vi "Begin.vi"(8 "error in":errorcluster) -> (0 "error out":errorcluster)   [LabVIEW 2019]
doc: "Called before other user functions, this VI is expected to open initial I/O refnums, load in file data, and do all program initialization. Notice that the <B>error out</B> terminal is simply used for data flow. Wiring it to other structures or subVIs ensures that this VI runs first."
uses:
  <vilib>/Rock Robotics/WPI/DriverStation/WPI_DriverStationRobotMode2.ctl
  <vilib>/Rock Robotics/WPI/ThirdParty/Phoenix-LabVIEW/Motor Controller/Controls/CTRE_Phoenix_MotorControl_ControlMode.ctl
  <vilib>/Rock Robotics/WPI/Solenoid/WPI_SolenoidChannel.ctl
  <vilib>/Rock Robotics/WPI/Joystick/WPI_JoystickDeviceEnum.ctl
  <vilib>/Rock Robotics/SystemInterfaces/DIO/FPGA_DIOPWMChannel.ctl
  <vilib>/Rock Robotics/SystemInterfaces/DIO/FPGA_DIOChannel.ctl
  <vilib>/Rock Robotics/WPI/ThirdParty/Phoenix-LabVIEW/Motor Controller/Controls/CTRE_Phoenix_MotorControl_FeedbackDevice.ctl
  <vilib>/Rock Robotics/WPI/SafetyOutput/WPI_SafetyOutputConfigMenu.ctl
  Robot Global Data.vi
  <vilib>/Rock Robotics/Network Tables/NT Write String Array.vi
  <vilib>/Rock Robotics/WPI/Solenoid/WPI_SolenoidOpenDouble.vi
  <vilib>/Rock Robotics/WPI/Switch/WPI_SwitchOpenLimit.vi
  <vilib>/Rock Robotics/WPI/MotorControl/WPI_MotorControlOpen SPARK.vi
  <vilib>/Rock Robotics/WPI/RobotDrive/WPI_RobotDriveOpen2MotorWithExistingMotors.vi
  <vilib>/Rock Robotics/WPI/MotorControl/WPI_MotorControlOpen VictorSP.vi
  <vilib>/Rock Robotics/WPI/RobotDrive/WPI_RobotDriveOpen2MotorWithTalon.vi
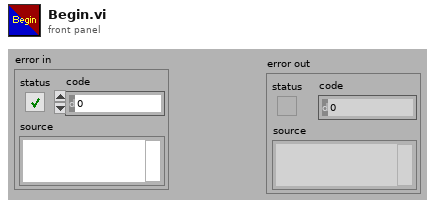
[diagram p1: front panel]
types:
  T1 = typedef "WPI_SafetyOutputConfigMenu.ctl" = enum16{"Enable", "Disable"}
  T2 = typedef "FPGA_DIOPWMChannel.ctl" = enum8{"PWM 0", "PWM 1", "PWM 2", "PWM 3", "PWM 4", "PWM 5", "PWM 6", "PWM 7", "PWM 8", "PWM 9", "PWM MXP 0", "PWM MXP 1", "PWM MXP 2", "PWM MXP 3", "PWM MXP 4", "PWM MXP 5", "PWM MXP 6", "PWM MXP 7", "PWM MXP 8", "PWM MXP 9", "Invalid"}
  T3 = typedef "WPI_JoystickDeviceEnum.ctl" = enum16{"USB 0", "USB 1", "USB 2", "USB 3", "USB 4", "USB 5"}
  T4 = typedef "CTRE_Phoenix_MotorControl_FeedbackDevice.ctl" = i8
  T5 = typedef "WPI_SolenoidChannel.ctl" = enum8{"Solenoid 0", "Solenoid 1", "Solenoid 2", "Solenoid 3", "Solenoid 4", "Solenoid 5", "Solenoid 6", "Solenoid 7", "Invalid"}
  T6 = typedef "CTRE_Phoenix_MotorControl_ControlMode.ctl" = u16
  T7 = typedef "FPGA_DIOChannel.ctl" = enum8{"DIO 0", "DIO 1", "DIO 2", "DIO 3", "DIO 4", "DIO 5", "DIO 6", "DIO 7", "DIO 8", "DIO 9", "DIO MXP 0", "DIO MXP 1", "DIO MXP 2", "DIO MXP 3", "DIO MXP 4", "DIO MXP 5", "DIO MXP 6", "DIO MXP 7", "DIO MXP 8", "DIO MXP 9", "DIO MXP 10", "DIO MXP 11", "DIO MXP 12", "DIO MXP 13", "DIO MXP 14", "DIO MXP 15", "SPI Port CS1", "SPI Port CS2", "SPI Port CS3", "SPI Port MISO", "SPI Port MOSI", "Invalid"}
  T8 = typedef "WPI_DriverStationRobotMode2.ctl" = enum16{"Autonomous Disabled", "Autonomous Enabled", "Teleop Disabled", "Teleop Enabled", "Disconnected", "Finish", "Test Disabled", "Test Enabled", "Emergency Stopped"}
  T9 = typedef "WPI_JoystickDevRef.ctl" = cluster{"Device":T3}
  T10 = typedef "WPI_RobotDriveDevRef.ctl" = cluster{"DevStatus":errorcluster, "Motors[]":T11[], "Square Inputs":bool, "Max Output":dbl}
  T11 = typedef "WPI_MotorControlDeviceRef.ctl" = cluster{"DeviceStatus":errorcluster, "Type":T12, "PWM":cluster{"PWM Channel":T2, "DeadBand":T13}, "CAN":cluster{"Device Number":u8, "SetOutput VI Ref":variant, "GetOutput VI Ref":variant, "Enable VI Ref":variant, "Disable VI Ref":variant, "Data":variant}, "Invert":bool, "DIO PWM":cluster{"PWM \"Enable\" Channel":T2, "DIOChannel":T7, "PWM Rate":dbl}}
  T12 = typedef "WPI_MotorControlType.ctl" = enum16{"PWM", "CAN", "DIO PWM"}
  T13 = typedef "WPI_PWMDeadband.ctl" = cluster{"Name":string, "maxPositivePwm":i32, "minPositivePwm":i32, "centerPwm":i32, "maxNegativePwm":i32, "minNegativePwm":i32, "angularRange":u16}
  T14 = typedef "WPI_ServoDeviceRef.ctl" = cluster{"DeviceStatus":errorcluster, "PWM Channel":T2, "DeadBand":T13}
  T15 = typedef "WPI_SwitchDevRef.ctl" = cluster{"DevStatus":errorcluster, "DIO Channel":T7, "CntIndex":T16, "Normally Closed":bool}
  T16 = typedef "FPGA_CounterCtrSystemIndex.ctl" = enum8{"Ctr 0", "Ctr 1", "Ctr 2", "Ctr 3", "Ctr 4", "Ctr 5", "Ctr 6", "Ctr 7", "Invalid"}
  T17 = typedef "WPI_SolenoidDevRef.ctl" = cluster{"DevStatus":errorcluster, "Pneumatics Control Module":u8, "Forward Solenoid Channel":T5, "Reverse Solenoid Channel":T5}
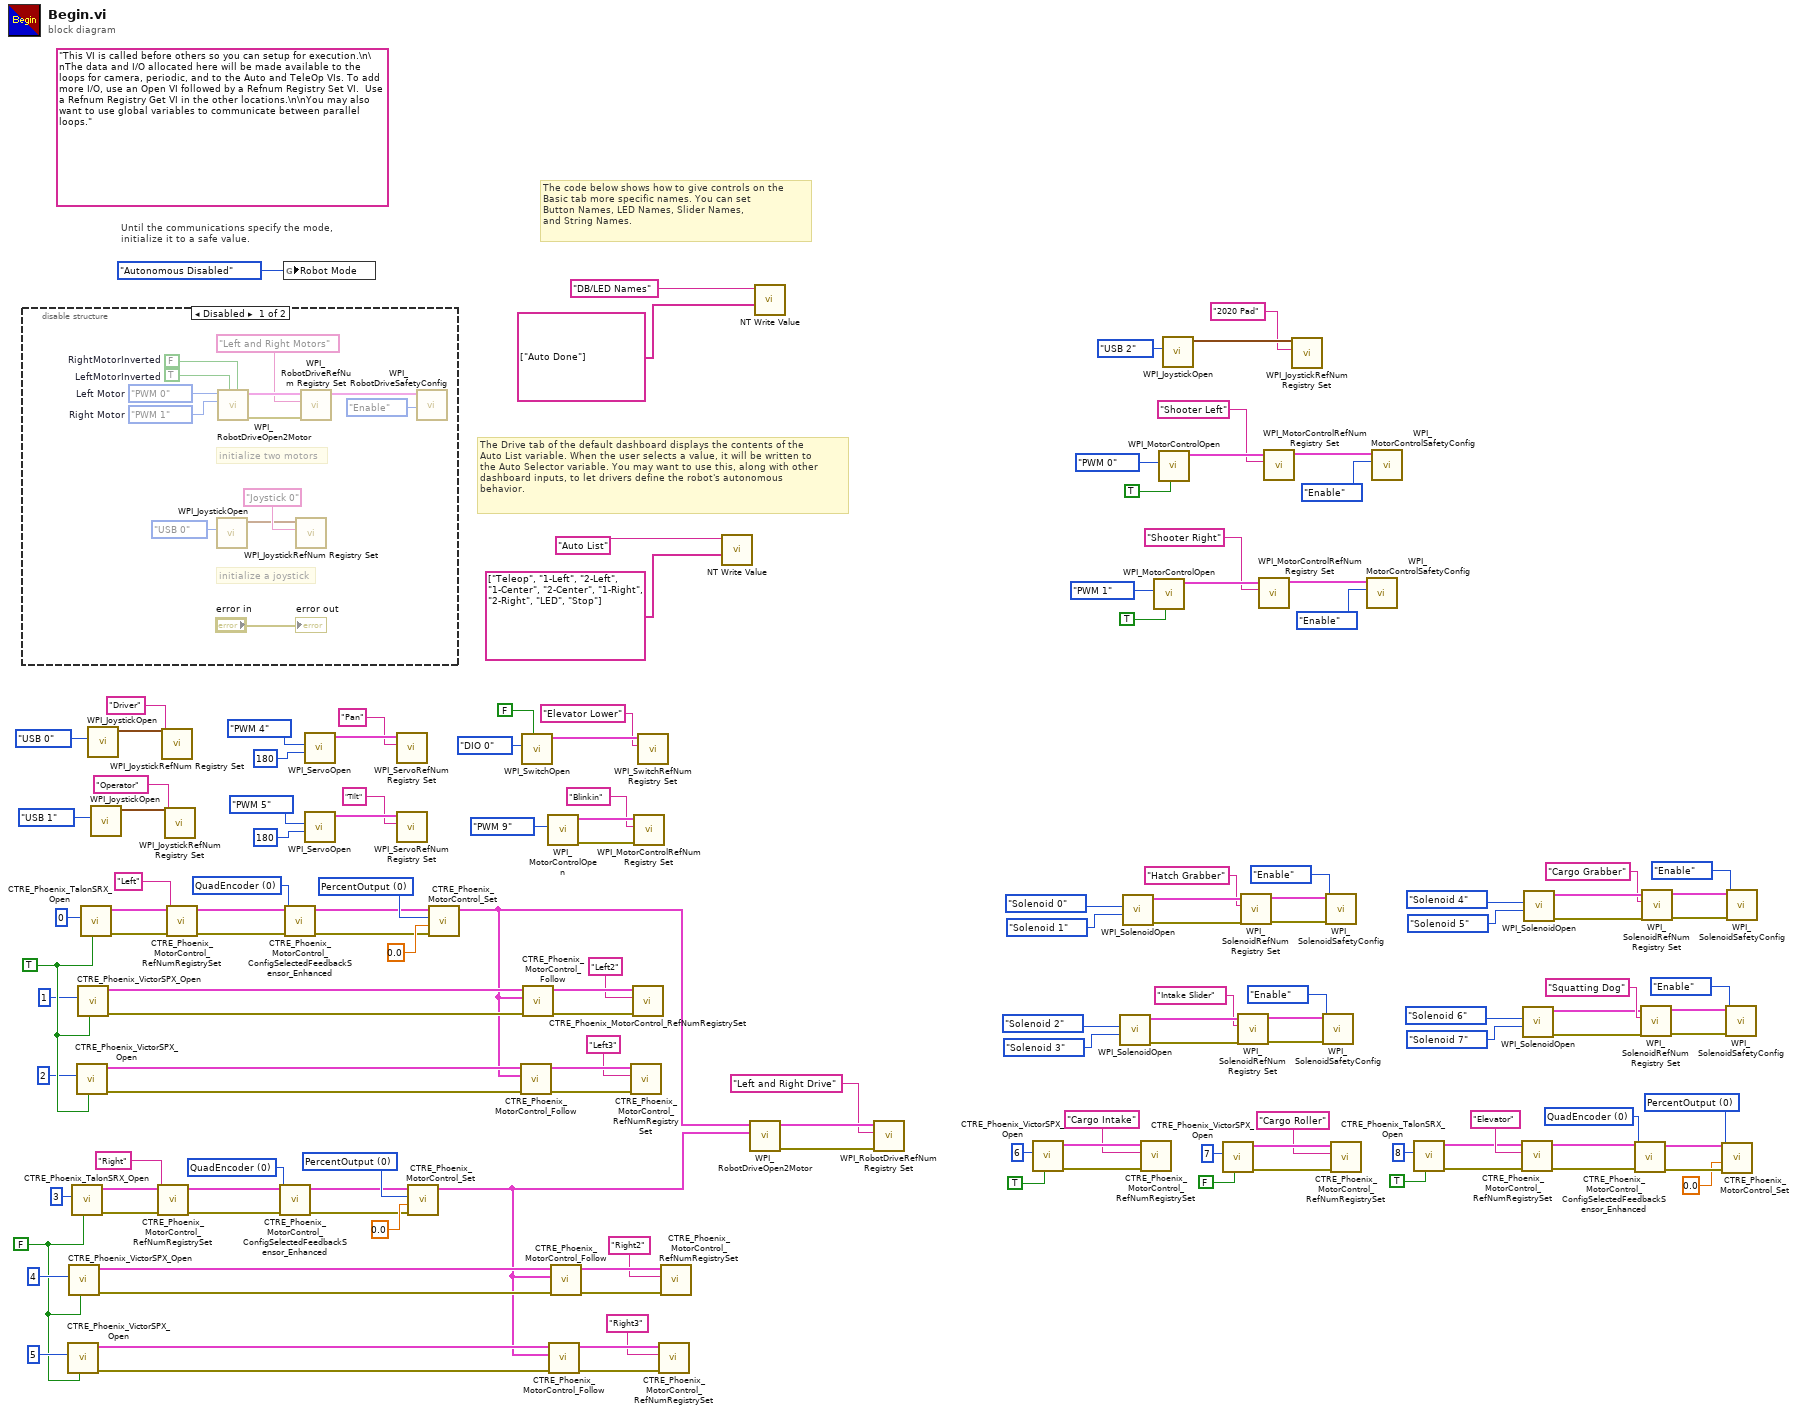
[diagram p0: block diagram]
diagram:
  w23 = T4 0 items=["QuadEncoder"=0, "Analog"=2, "Tachometer"=4, "Pulse Width Encoded Position"=8, "Sensor Sum (S0 + S1)"=9, "Sensor Difference (D0 - D1)"=10, "Remote Source 0"=11, "Remote Source 1"=12, "Software Emulated"=15] ("Feedback Device")
  w27 = T4 0 items=["QuadEncoder"=0, "Analog"=2, "Tachometer"=4, "Pulse Width Encoded Position"=8, "Sensor Sum (S0 + S1)"=9, "Sensor Difference (D0 - D1)"=10, "Remote Source 0"=11, "Remote Source 1"=12, "Software Emulated"=15] ("Feedback Device")
  w44 = T6 0 items=["PercentOutput"=0, "Position"=1, "Velocity"=2, "Current"=3, "Follower"=5, "MotionProfile"=6, "MotionMagic"=7, "MotionProfileArc"=10, "Disabled"=15] ("Control Mode")
  w47 = T4 0 items=["QuadEncoder"=0, "Analog"=2, "Tachometer"=4, "Pulse Width Encoded Position"=8, "Sensor Sum (S0 + S1)"=9, "Sensor Difference (D0 - D1)"=10, "Remote Source 0"=11, "Remote Source 1"=12, "Software Emulated"=15] ("Feedback Device")
  w110 = T6 0 items=["PercentOutput"=0, "Position"=1, "Velocity"=2, "Current"=3, "Follower"=5, "MotionProfile"=6, "MotionMagic"=7, "MotionProfileArc"=10, "Disabled"=15] ("Control Mode")
  w111 = T6 0 items=["PercentOutput"=0, "Position"=1, "Velocity"=2, "Current"=3, "Follower"=5, "MotionProfile"=6, "MotionMagic"=7, "MotionProfileArc"=10, "Disabled"=15] ("Control Mode")
  w70 = FALSE ("Invert")
  w142 = TRUE ("Invert")
  (unwired) "This VI is called before others so you can setup for execution.\n\nThe data and I/O allocated here will be made available to the loops for camera, periodic, and to the Auto and TeleOp VIs. To add more I/O, use an Open VI followed by a Refnum Registry Set VI.  Use a Refnum Registry Get VI in the other locations.\n\nYou may also want to use global variables to communicate between parallel loops."
  # "The Drive tab of the default dashboard displays the contents of the\nAuto List variable. When the user selects a value, it will be written to\nthe Auto Selector variable. You may want to use this, along with other\ndashboard inputs, to let drivers define the robot's autonomous\nbehavior."
  # "The code below shows how to give controls on the\nBasic tab more specific names. You can set\nButton Names, LED Names, Slider Names,\nand String Names."
  # "Until the communications specify the mode,\ninitialize it to a safe value."
  n1 = disable-structure shown="Disabled" {
    frame Disabled {
      w156 = FPGA_DIOPWMChannel."PWM 1"  # Right Motor
      w157 = FPGA_DIOPWMChannel."PWM 0"  # Left Motor
      w161 = TRUE  # LeftMotorInverted
      w162 = FALSE  # RightMotorInverted
      # "initialize a joystick"
      # "initialize two motors"
      n2 = call <vilib>:"WPI_JoystickOpen.vi"("JoystickDevice"=WPI_JoystickDeviceEnum."USB 0") -> ("JoystickDevRef"=w152:T9)  [unwired: 10 in]
      n3 = call-poly <vilib>:"WPI_RobotDriveOpen2Motor.vi"("Right Motor Inverted"=w162, "Left Motor Inverted"=w161, "Right Motor"=w156, "Left Motor"=w157) -> ("error out"=w158:errorcluster, "RobotDriveDevRef"=w160:T10)  [unwired: 1 in, 5 out]
      n4 = call <vilib>:"WPI_JoystickRefNum Registry Set.vi"("refnum name"="Joystick 0", "JoystickDevRef"=w152) -> ()  [unwired: 8 in, 2 out]
      n5 = call <vilib>:"WPI_RobotDriveRefNum Registry Set.vi"("error in (no error)"=w158, "refnum name"="Left and Right Motors", "RobotDriveDevRef"=w160) -> ("RobotDriveDevRef"=w155:T10)  [unwired: 1 in, 7 out]
      n6 = call <vilib>:"WPI_RobotDriveSafetyConfig.vi"("mode"=WPI_SafetyOutputConfigMenu."Enable", "RobotDriveDevRef"=w155) -> ()  [unwired: 8 in, 2 out]
      "error out" <- "error in"
    }
    frame Enabled {
    }
  }
  n7 = call <vilib>:"CTRE_Phoenix_VictorSPX_Open.vi"("Invert"=w70, "Device Number"=u8 5) -> ("error out"=w119:errorcluster, "CAN Talon SRX Ref"=w123:T11)  [unwired: 8 in]
  n8 = call <vilib>:"CTRE_Phoenix_VictorSPX_Open.vi"("Invert"=w70, "Device Number"=u8 4) -> ("error out"=w121:errorcluster, "CAN Talon SRX Ref"=w128:T11)  [unwired: 8 in]
  n9 = call <vilib>:"CTRE_Phoenix_TalonSRX_Open.vi"("Invert"=w70, "Device Number"=u8 3) -> ("error out"=w122:errorcluster, "CAN Talon SRX Ref"=w130:T11)  [unwired: 8 in]
  n10 = call <vilib>:"CTRE_Phoenix_VictorSPX_Open.vi"("Invert"=w142, "Device Number"=u8 2) -> ("error out"=w132:errorcluster, "CAN Talon SRX Ref"=w136:T11)  [unwired: 8 in]
  n11 = call <vilib>:"CTRE_Phoenix_VictorSPX_Open.vi"("Invert"=w142, "Device Number"=u8 1) -> ("error out"=w134:errorcluster, "CAN Talon SRX Ref"=w141:T11)  [unwired: 8 in]
  n12 = call <vilib>:"CTRE_Phoenix_TalonSRX_Open.vi"("Invert"=w142, "Device Number"=u8 0) -> ("error out"=w135:errorcluster, "CAN Talon SRX Ref"=w144:T11)  [unwired: 8 in]
  n13 = call <vilib>:"WPI_JoystickOpen.vi"("JoystickDevice"=WPI_JoystickDeviceEnum."USB 0") -> ("JoystickDevRef"=w53:T9)  [unwired: 10 in]
  n14 = call <vilib>:"WPI_JoystickOpen.vi"("JoystickDevice"=WPI_JoystickDeviceEnum."USB 1") -> ("JoystickDevRef"=w83:T9)  [unwired: 10 in]
  n15 = call <vilib>:"CTRE_Phoenix_MotorControl_RefNumRegistrySet.vi"("error in (no error)"=w122, "refnum name"="Right", "PhoenixMotorControlDevRef"=w130) -> ("error out"=w21:errorcluster, "PhoenixMotorControlDevRef"=w16:T11)  [unwired: 7 in]
  n16 = call <vilib>:"WPI_JoystickRefNum Registry Set.vi"("refnum name"="Driver", "JoystickDevRef"=w53) -> ()  [unwired: 8 in, 2 out]
  n17 = call <vilib>:"WPI_JoystickRefNum Registry Set.vi"("refnum name"="Operator", "JoystickDevRef"=w83) -> ()  [unwired: 8 in, 2 out]
  n18 = call <vilib>:"CTRE_Phoenix_MotorControl_RefNumRegistrySet.vi"("error in (no error)"=w135, "refnum name"="Left", "PhoenixMotorControlDevRef"=w144) -> ("error out"=w26:errorcluster, "PhoenixMotorControlDevRef"=w17:T11)  [unwired: 7 in]
  n19 = call <vilib>:"CTRE_Phoenix_MotorControl_ConfigSelectedFeedbackSensor_Enhanced.vi"("error in (no error)"=w21, "Feedback Device"=w23, "PhoenixMotorControlDevRef"=w16) -> ("error out"=w20:errorcluster, "PhoenixMotorControlDevRef"=w22:T11)  [unwired: 7 in]
  n20 = global write "Robot Global Data.vi" "Robot Mode"(WPI_DriverStationRobotMode2."Autonomous Disabled" ("Robot Mode")) -> ()
  n21 = call <vilib>:"CTRE_Phoenix_MotorControl_ConfigSelectedFeedbackSensor_Enhanced.vi"("error in (no error)"=w26, "Feedback Device"=w27, "PhoenixMotorControlDevRef"=w17) -> ("error out"=w24:errorcluster, "PhoenixMotorControlDevRef"=w25:T11)  [unwired: 7 in]
  n22 = call <vilib>:"WPI_ServoOpen.vi"("Angular Range"=u16 180, "PWM Channel"=FPGA_DIOPWMChannel."PWM 4") -> ("ServoDeviceRef"=w79:T14)  [unwired: 8 in, 1 out]
  n23 = call <vilib>:"WPI_ServoOpen.vi"("Angular Range"=u16 180, "PWM Channel"=FPGA_DIOPWMChannel."PWM 5") -> ("ServoDeviceRef"=w76:T14)  [unwired: 8 in, 1 out]
  n24 = call <vilib>:"WPI_ServoRefNum Registry Set.vi"("refnum name"="Pan", "ServoDeviceRef"=w79) -> ()  [unwired: 8 in, 2 out]
  n25 = call <vilib>:"WPI_ServoRefNum Registry Set.vi"("refnum name"="Tilt", "ServoDeviceRef"=w76) -> ()  [unwired: 8 in, 2 out]
  n26 = call <vilib>:"CTRE_Phoenix_MotorControl_Set.vi"("error in (no error)"=w20, "Output"=0.0, "Control Mode"=w110, "PhoenixMotorControlDevRef"=w22) -> ("PhoenixMotorControlDevRef"=w18:T11)  [unwired: 6 in, 1 out]
  n27 = call <vilib>:"CTRE_Phoenix_MotorControl_Set.vi"("error in (no error)"=w24, "Output"=0.0, "Control Mode"=w111, "PhoenixMotorControlDevRef"=w25) -> ("PhoenixMotorControlDevRef"=w19:T11)  [unwired: 6 in, 1 out]
  n28 = call <vilib>:"CTRE_Phoenix_MotorControl_Follow.vi"("error in (no error)"=w132, "Master Controller to Follow"=w19, "PhoenixMotorControlDevRef"=w136) -> ("error out"=w131:errorcluster, "PhoenixMotorControlDevRef"=w138:T11)  [unwired: 7 in]
  n29 = call-poly <vilib>:"WPI_SwitchOpen.vi"("Normally Closed"=FALSE, "DIO Channel"=FPGA_DIOChannel."DIO 0") -> ("SwitchDevRef"=w72:T15)  [unwired: 8 in, 1 out]
  n30 = call <vilib>:"CTRE_Phoenix_MotorControl_Follow.vi"("error in (no error)"=w134, "Master Controller to Follow"=w19, "PhoenixMotorControlDevRef"=w141) -> ("error out"=w133:errorcluster, "PhoenixMotorControlDevRef"=w140:T11)  [unwired: 7 in]
  n31 = call-poly <vilib>:"WPI_MotorControlOpen.vi"("PWM Channel"=FPGA_DIOPWMChannel."PWM 9") -> ("error out"=w37:errorcluster, "MotorControlDeviceRef"=w39:T11)  [unwired: 9 in]
  n32 = call <vilib>:"CTRE_Phoenix_MotorControl_Follow.vi"("error in (no error)"=w119, "Master Controller to Follow"=w18, "PhoenixMotorControlDevRef"=w123) -> ("error out"=w118:errorcluster, "PhoenixMotorControlDevRef"=w125:T11)  [unwired: 7 in]
  n33 = call <vilib>:"CTRE_Phoenix_MotorControl_Follow.vi"("error in (no error)"=w121, "Master Controller to Follow"=w18, "PhoenixMotorControlDevRef"=w128) -> ("error out"=w120:errorcluster, "PhoenixMotorControlDevRef"=w127:T11)  [unwired: 7 in]
  n34 = call <vilib>:"CTRE_Phoenix_MotorControl_RefNumRegistrySet.vi"("error in (no error)"=w131, "refnum name"="Left3", "PhoenixMotorControlDevRef"=w138) -> ()  [unwired: 7 in, 2 out]
  n35 = call <vilib>:"CTRE_Phoenix_MotorControl_RefNumRegistrySet.vi"("error in (no error)"=w133, "refnum name"="Left2", "PhoenixMotorControlDevRef"=w140) -> ()  [unwired: 7 in, 2 out]
  n36 = call <vilib>:"WPI_MotorControlRefNum Registry Set.vi"("error in (no error)"=w37, "refnum name"="Blinkin", "MotorControlDevRef"=w39) -> ()  [unwired: 7 in, 2 out]
  n37 = call <vilib>:"WPI_SwitchRefNum Registry Set.vi"("refnum name"="Elevator Lower", "SwitchDevRef"=w72) -> ()  [unwired: 8 in, 2 out]
  n38 = call <vilib>:"CTRE_Phoenix_MotorControl_RefNumRegistrySet.vi"("error in (no error)"=w118, "refnum name"="Right3", "PhoenixMotorControlDevRef"=w125) -> ()  [unwired: 7 in, 2 out]
  n39 = call <vilib>:"CTRE_Phoenix_MotorControl_RefNumRegistrySet.vi"("error in (no error)"=w120, "refnum name"="Right2", "PhoenixMotorControlDevRef"=w127) -> ()  [unwired: 7 in, 2 out]
  n40 = call-poly <vilib>:"NT Write Value.vi"("String Array"=string[] ["Teleop", "1-Left", "2-Left", "1-Center", "2-Center", "1-Right", "2-Right", "LED", "Stop"], "Name"="Auto List") -> ()  [unwired: 9 in, 1 out]
  n41 = call-poly <vilib>:"WPI_RobotDriveOpen2Motor.vi"("Right Motor Dev Ref"=w18, "Left Motor Dev Ref"=w19) -> ("error out"=w50:errorcluster, "RobotDriveDevRef"=w52:T10)  [unwired: 8 in]
  n42 = call-poly <vilib>:"NT Write Value.vi"("String Array"=string[] ["Auto Done"], "Name"="DB/LED Names") -> ()  [unwired: 9 in, 1 out]
  n43 = call <vilib>:"WPI_RobotDriveRefNum Registry Set.vi"("error in (no error)"=w50, "refnum name"="Left and Right Drive", "RobotDriveDevRef"=w52) -> ()  [unwired: 7 in, 2 out]
  n44 = call <vilib>:"CTRE_Phoenix_VictorSPX_Open.vi"("Invert"=TRUE, "Device Number"=u8 6) -> ("error out"=w67:errorcluster, "CAN Talon SRX Ref"=w68:T11)  [unwired: 8 in]
  n45 = call-poly <vilib>:"WPI_SolenoidOpen.vi"("Reverse Solenoid Channel"=WPI_SolenoidChannel."Solenoid 3", "Forward Solenoid Channel"=WPI_SolenoidChannel."Solenoid 2") -> ("error out"=w95:errorcluster, "SolenoidDevRef"=w97:T17)  [unwired: 8 in]
  n46 = call-poly <vilib>:"WPI_SolenoidOpen.vi"("Reverse Solenoid Channel"=WPI_SolenoidChannel."Solenoid 1", "Forward Solenoid Channel"=WPI_SolenoidChannel."Solenoid 0") -> ("error out"=w103:errorcluster, "SolenoidDevRef"=w105:T17)  [unwired: 8 in]
  n47 = call <vilib>:"CTRE_Phoenix_MotorControl_RefNumRegistrySet.vi"("error in (no error)"=w67, "refnum name"="Cargo Intake", "PhoenixMotorControlDevRef"=w68) -> ()  [unwired: 7 in, 2 out]
  n48 = call-poly <vilib>:"WPI_MotorControlOpen.vi"("Invert"=TRUE, "PWM Channel"=FPGA_DIOPWMChannel."PWM 1") -> ("MotorControlDeviceRef"=w6:T11)  [unwired: 8 in, 1 out]
  n49 = call-poly <vilib>:"WPI_MotorControlOpen.vi"("Invert"=TRUE, "PWM Channel"=FPGA_DIOPWMChannel."PWM 0") -> ("MotorControlDeviceRef"=w11:T11)  [unwired: 8 in, 1 out]
  n50 = call <vilib>:"WPI_JoystickOpen.vi"("JoystickDevice"=WPI_JoystickDeviceEnum."USB 2") -> ("JoystickDevRef"=w14:T9)  [unwired: 10 in]
  n51 = call <vilib>:"CTRE_Phoenix_VictorSPX_Open.vi"("Invert"=FALSE, "Device Number"=u8 7) -> ("error out"=w63:errorcluster, "CAN Talon SRX Ref"=w64:T11)  [unwired: 8 in]
  n52 = call <vilib>:"WPI_SolenoidRefNum Registry Set.vi"("error in (no error)"=w95, "refnum name"="Intake Slider", "SolenoidDevRef"=w97) -> ("error out"=w93:errorcluster, "SolenoidDevRef"=w94:T17)  [unwired: 7 in]
  n53 = call <vilib>:"WPI_SolenoidRefNum Registry Set.vi"("error in (no error)"=w103, "refnum name"="Hatch Grabber", "SolenoidDevRef"=w105) -> ("error out"=w101:errorcluster, "SolenoidDevRef"=w102:T17)  [unwired: 7 in]
  n54 = call <vilib>:"WPI_MotorControlRefNum Registry Set.vi"("refnum name"="Shooter Right", "MotorControlDevRef"=w6) -> ("MotorControlDevRef"=w4:T11)  [unwired: 8 in, 1 out]
  n55 = call <vilib>:"WPI_MotorControlRefNum Registry Set.vi"("refnum name"="Shooter Left", "MotorControlDevRef"=w11) -> ("MotorControlDevRef"=w9:T11)  [unwired: 8 in, 1 out]
  n56 = call <vilib>:"WPI_JoystickRefNum Registry Set.vi"("refnum name"="2020 Pad", "JoystickDevRef"=w14) -> ()  [unwired: 8 in, 2 out]
  n57 = call <vilib>:"WPI_SolenoidSafetyConfig.vi"("error in (no error)"=w93, "mode"=WPI_SafetyOutputConfigMenu."Enable", "SolenoidDevRef"=w94) -> ()  [unwired: 7 in, 2 out]
  n58 = call <vilib>:"WPI_SolenoidSafetyConfig.vi"("error in (no error)"=w101, "mode"=WPI_SafetyOutputConfigMenu."Enable", "SolenoidDevRef"=w102) -> ()  [unwired: 7 in, 2 out]
  n59 = call <vilib>:"CTRE_Phoenix_MotorControl_RefNumRegistrySet.vi"("error in (no error)"=w63, "refnum name"="Cargo Roller", "PhoenixMotorControlDevRef"=w64) -> ()  [unwired: 7 in, 2 out]
  n60 = call <vilib>:"WPI_MotorControlSafetyConfig.vi"("mode"=WPI_SafetyOutputConfigMenu."Enable", "MotorControlDevRef"=w4) -> ()  [unwired: 8 in, 2 out]
  n61 = call <vilib>:"WPI_MotorControlSafetyConfig.vi"("mode"=WPI_SafetyOutputConfigMenu."Enable", "MotorControlDevRef"=w9) -> ()  [unwired: 8 in, 2 out]
  n62 = call <vilib>:"CTRE_Phoenix_TalonSRX_Open.vi"("Invert"=TRUE, "Device Number"=u8 8) -> ("error out"=w58:errorcluster, "CAN Talon SRX Ref"=w57:T11)  [unwired: 8 in]
  n63 = call <vilib>:"CTRE_Phoenix_MotorControl_RefNumRegistrySet.vi"("error in (no error)"=w58, "refnum name"="Elevator", "PhoenixMotorControlDevRef"=w57) -> ("error out"=w48:errorcluster, "PhoenixMotorControlDevRef"=w49:T11)  [unwired: 7 in]
  n64 = call-poly <vilib>:"WPI_SolenoidOpen.vi"("Reverse Solenoid Channel"=WPI_SolenoidChannel."Solenoid 7", "Forward Solenoid Channel"=WPI_SolenoidChannel."Solenoid 6") -> ("error out"=w33:errorcluster, "SolenoidDevRef"=w31:T17)  [unwired: 8 in]
  n65 = call-poly <vilib>:"WPI_SolenoidOpen.vi"("Reverse Solenoid Channel"=WPI_SolenoidChannel."Solenoid 5", "Forward Solenoid Channel"=WPI_SolenoidChannel."Solenoid 4") -> ("error out"=w87:errorcluster, "SolenoidDevRef"=w89:T17)  [unwired: 8 in]
  n66 = call <vilib>:"CTRE_Phoenix_MotorControl_ConfigSelectedFeedbackSensor_Enhanced.vi"("error in (no error)"=w48, "Feedback Device"=w47, "PhoenixMotorControlDevRef"=w49) -> ("error out"=w45:errorcluster, "PhoenixMotorControlDevRef"=w46:T11)  [unwired: 7 in]
  n67 = call <vilib>:"WPI_SolenoidRefNum Registry Set.vi"("error in (no error)"=w33, "refnum name"="Squatting Dog", "SolenoidDevRef"=w31) -> ("error out"=w35:errorcluster, "SolenoidDevRef"=w34:T17)  [unwired: 7 in]
  n68 = call <vilib>:"WPI_SolenoidRefNum Registry Set.vi"("error in (no error)"=w87, "refnum name"="Cargo Grabber", "SolenoidDevRef"=w89) -> ("error out"=w85:errorcluster, "SolenoidDevRef"=w86:T17)  [unwired: 7 in]
  n69 = call <vilib>:"CTRE_Phoenix_MotorControl_Set.vi"("error in (no error)"=w45, "Output"=0.0, "Control Mode"=w44, "PhoenixMotorControlDevRef"=w46) -> ()  [unwired: 6 in, 2 out]
  n70 = call <vilib>:"WPI_SolenoidSafetyConfig.vi"("error in (no error)"=w35, "mode"=WPI_SafetyOutputConfigMenu."Enable", "SolenoidDevRef"=w34) -> ()  [unwired: 7 in, 2 out]
  n71 = call <vilib>:"WPI_SolenoidSafetyConfig.vi"("error in (no error)"=w85, "mode"=WPI_SafetyOutputConfigMenu."Enable", "SolenoidDevRef"=w86) -> ()  [unwired: 7 in, 2 out]
